vi "Swerve Drive Brushless V2.vi"(0 "Front Left Offset":dbl, 1 "Direction":T6, 5 "Front Right Offset":dbl, 7 "Align 90":bool, 9 "Back Left  Offset":dbl, 10 "Wheel Base Length":dbl=20.0, 11 "Back Right Offset":dbl, 12 "Drive Commands":T5, 15 "Wheel Base Width":dbl=23.0) -> (2 "Front Left Drive Output":T1, 3 "Front Right Drive Output":T3, 13 "Back Left Drive Output":T2, 14 "Back Right Drive Output":T4)   [LabVIEW 2020]
uses:
  Direction Commands.ctl
  Drive Comands.ctl
  Back Left Outputctl.ctl
  Front Right Output.ctl
  Back Right Output.ctl
  Front Left Output.ctl
panel:
  in  "Front Left Drive Output":T1
  in  "Back Right Drive Output":T4
  in  "Right  Front Drive Output":T3
  in  "Back Left Drive Output":T2
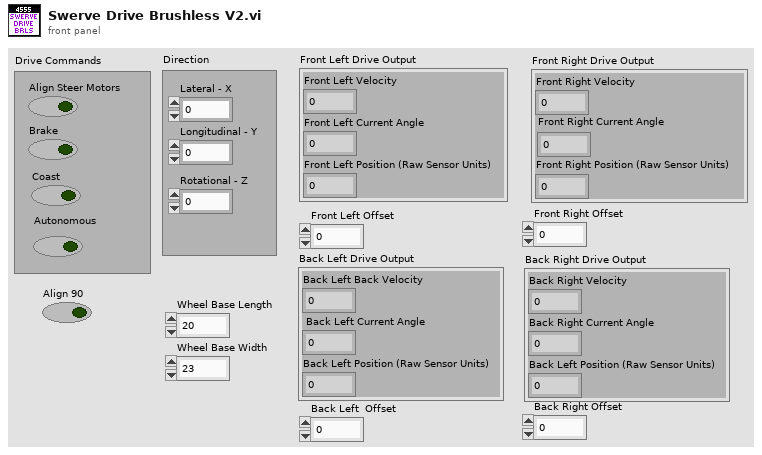
[diagram p1: front panel]
types:
  T1 = typedef "Front Left Output.ctl" = cluster{"Front Left Velocity":dbl, "Front Left Current Angle":dbl, "Front Left Position (Raw Sensor Units)":i32}
  T2 = typedef "Back Left Outputctl.ctl" = cluster{"Back Left Back Velocity":dbl, " Back Left Current Angle":dbl, "Back Left Position (Raw Sensor Units)":i32}
  T3 = typedef "Front Right Output.ctl" = cluster{"Front Right Velocity":dbl, "Front Right Current Angle":dbl, "Front Right Position (Raw Sensor Units)":i32}
  T4 = typedef "Back Right Output.ctl" = cluster{"Back Right Velocity":dbl, "Back Right Current Angle":dbl, "Back Left Position (Raw Sensor Units)":i32}
  T5 = typedef "Drive Comands.ctl" = cluster{"Align Steer Motors":bool, "Brake":bool, "Coast":bool, "Autonomous":bool}
  T6 = typedef "Direction Commands.ctl" = cluster{"Lateral - X":dbl, "Longitudinal - Y":dbl, "Rotational - Z":dbl}
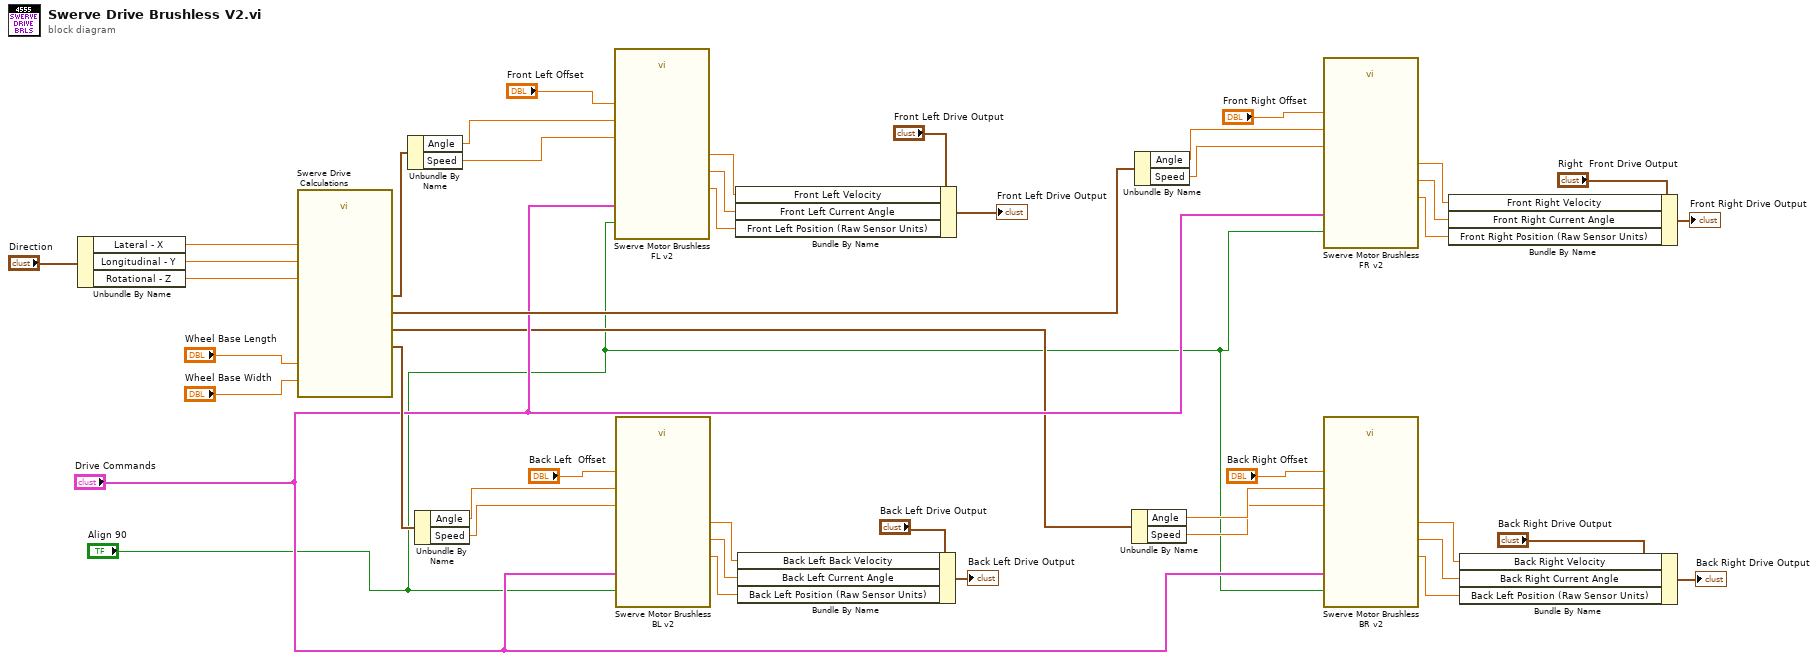
[diagram p0: block diagram]
diagram:
  n1 = Unbundle By Name("Direction") -> ("Lateral - X"=w37:dbl, "Longitudinal - Y"=w36:dbl, "Rotational - Z"=w40:dbl)
  n2 = call "Swerve Drive Calculations.vi"("Wheel Base Width"="Wheel Base Width", "Wheel Base Length"="Wheel Base Length", "Longitudinal - Y"=w36, "Rotational - Z"=w40, "Lateral - X"=w37) -> ("Back Right Drive"=w38:cluster{"Speed":dbl, "Angle":dbl}, "Back Left Drive"=w44:cluster{"Speed":dbl, "Angle":dbl}, "Front Right Drive"=w43:cluster{"Speed":dbl, "Angle":dbl}, "Front Left  Drive"=w42:cluster{"Speed":dbl, "Angle":dbl})  [unwired: 1 in]
  n3 = Unbundle By Name(w42) -> ("Angle"=w35:dbl, "Speed"=w30:dbl)
  n4 = Unbundle By Name(w44) -> ("Angle"=w19:dbl, "Speed"=w18:dbl)
  n5 = call "Swerve Motor Brushless FL v2.vi"("Offset"="Front Left Offset", "Drive Commands"="Drive Commands", "Direction command (deg)"=w35, "Speed command"=w30, "Align 90"="Align 90") -> ("Front Left Position"=w31:dbl, "Front Left Current Angle"=w32:dbl, "Front Left Velocity"=w33:dbl)  [unwired: 2 in]
  n6 = call "Swerve Motor Brushless BL v2.vi"("Offset"="Back Left  Offset", "Drive Commands"="Drive Commands", "Direction command (deg)"=w19, "Speed command"=w18, "Align 90"="Align 90") -> ("Back Left Position"=w13:dbl, "Back Left Current Angle"=w14:dbl, "Back Left Velocity"=w16:dbl)  [unwired: 2 in]
  n7 = Bundle By Name(cluster="Front Left Drive Output", "Front Left Velocity"=w33, "Front Left Current Angle"=w32, "Front Left Position (Raw Sensor Units)"=w31) -> (→"Front Left Drive Output":T1)
  n8 = Bundle By Name(cluster="Back Left Drive Output", "Back Left Back Velocity"=w16, "Back Left Current Angle"=w14, "Back Left Position (Raw Sensor Units)"=w13) -> (→"Back Left Drive Output":T2)
  n9 = Unbundle By Name(w38) -> ("Angle"=w11:dbl, "Speed"=w10:dbl)
  n10 = Unbundle By Name(w43) -> ("Angle"=w27:dbl, "Speed"=w26:dbl)
  n11 = call "Swerve Motor Brushless FR v2.vi"("Offset"="Front Right Offset", "Drive Commands"="Drive Commands", "Direction command (deg)"=w27, "Speed command"=w26, "Align 90"="Align 90") -> ("Front Right Position"=w22:dbl, "Front Right Current Angle"=w21:dbl, "Front Right Velocity"=w23:dbl)  [unwired: 2 in]
  n12 = call "Swerve Motor Brushless BR v2.vi"("Offset"="Back Right Offset", "Drive Commands"="Drive Commands", "Direction command (deg)"=w11, "Speed command"=w10, "Align 90"="Align 90") -> ("Back Right Position"=w5:dbl, "Back Right Current Angle"=w6:dbl, "Back Right Velocity"=w7:dbl)  [unwired: 2 in]
  n13 = Bundle By Name(cluster="Right  Front Drive Output", "Front Right Velocity"=w23, "Front Right Current Angle"=w21, "Front Right Position (Raw Sensor Units)"=w22) -> (→"Front Right Drive Output":T3)
  n14 = Bundle By Name(cluster="Back Right Drive Output", "Back Right Velocity"=w7, "Back Right Current Angle"=w6, "Back Left Position (Raw Sensor Units)"=w5) -> (→"Back Right Drive Output":T4)
